vi "CrossbowWinch.vi"(10 "Buttons[5]":bool, 11 "Buttons[4]":bool) -> (2 "Output 2":dbl)   [LabVIEW 2014]
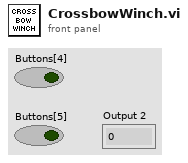
[diagram p1: front panel]
types:
  T1 = typedef "WPI_SwitchDevRef.ctl" = cluster{"DevStatus":errorcluster, "DIO Channel":T2, "Controller":T3, "CntIndex":T4, "Normally Closed":bool}
  T2 = typedef "FPGA_DIOChannel.ctl" = enum8{"DIO 0", "DIO 1", "DIO 2", "DIO 3", "DIO 4", "DIO 5", "DIO 6", "DIO 7", "DIO 8", "DIO 9", "DIO MXP 0", "DIO MXP 1", "DIO MXP 2", "DIO MXP 3", "DIO MXP 4", "DIO MXP 5", "DIO MXP 6", "DIO MXP 7", "DIO MXP 8", "DIO MXP 9", "DIO MXP 10", "DIO MXP 11", "DIO MXP 12", "DIO MXP 13", "DIO MXP 14", "DIO MXP 15", "Invalid"}
  T3 = typedef "FPGA_TypedefDigitalModule.ctl" = enum16{"Controller 1"}
  T4 = typedef "FPGA_CounterCtrSystemIndex.ctl" = enum8{"Ctr 0", "Ctr 1", "Ctr 2", "Ctr 3", "Ctr 4", "Ctr 5", "Ctr 6", "Ctr 7", "Invalid"}
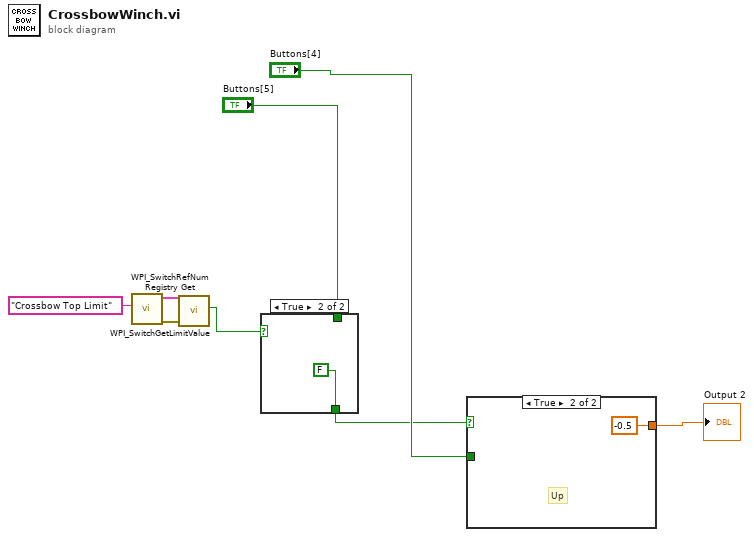
[diagram p0: block diagram]
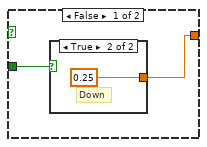
[diagram p3: hidden frame]
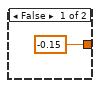
[diagram p4: hidden frame]
diagram:
  n1 = call <vilib>:"WPI_SwitchRefNum Registry Get.vi"("refnum name"="Crossbow Top Limit") -> ("error out"=w6:errorcluster, "SwitchDevRef"=w5:T1)  [unwired: 9 in]
  n2 = call <vilib>:"WPI_SwitchGetLimitValue.vi"("error in (no error)"=w6, "SwitchDevRef"=w5) -> ("Switch Pressed"=w3:bool)  [unwired: 7 in, 2 out]
  n3 = case shown="True" w3 {
    tunnel: [w9 FALSE] -> w2
    tunnel: "Buttons[5]" -> [w9 _]
    frame False {
    }
    frame True {
    }
  }
  n4 = case shown="True" w2 {
    tunnel: [w12 -0.5 ("Output")] -> w8
    tunnel: "Buttons[4]" -> [w11 _]
    frame False {
      n5 = case shown="True" w11 {
        tunnel: [-0.15 ("Output") 0.25 ("Output")] -> w12
        frame False {
        }
        frame True {
          # "Down"
        }
      }
    }
    frame True {
      # "Up"
    }
  }
  "Output 2" <- w8
